vi "write16bit3DFITS.vi"(2 "u16 pixmap":u16[][][](array[numeric])=array1x300x256[76800 elements], 3 "Text":string, 4 "file path":path=path "D:/temp/fitstest.fits") -> (0 "error out":errorcluster)   [LabVIEW 2011]
panel:
  out "FITS":T1={"BITPIX"=16.0, "NAXIS"=3.0, "NAXIS1"=300.0, "NAXIS2"=300.0, "NAXIS3"=1.0, "BZERO"=0.0, "BSCALE"=1.0}
  # "OK geht mit u16 daten"
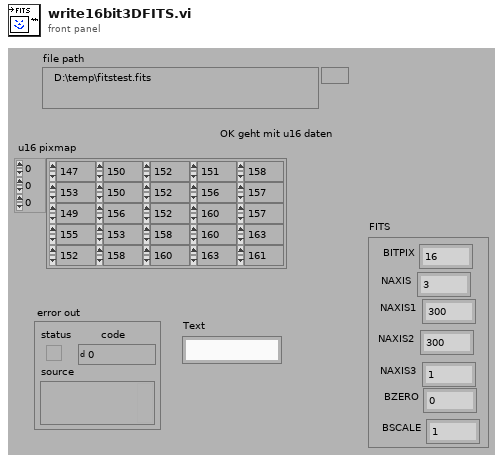
[diagram p1: front panel]
types:
  T1 = cluster{"BITPIX":sgl, "NAXIS":sgl, "NAXIS1":sgl, "NAXIS2":sgl, "NAXIS3":sgl, "BZERO":sgl, "BSCALE":sgl}
  T2 = cluster{"Tiff refnum":refnum<file>, "Byte-Reihenfolge (0:Big-Endian, 2:LSB)":enum16{"big-endian, network order", "native, host order", "little-endian"}}
  T3 = enum16{"big-endian, network order", "native, host order", "little-endian"}
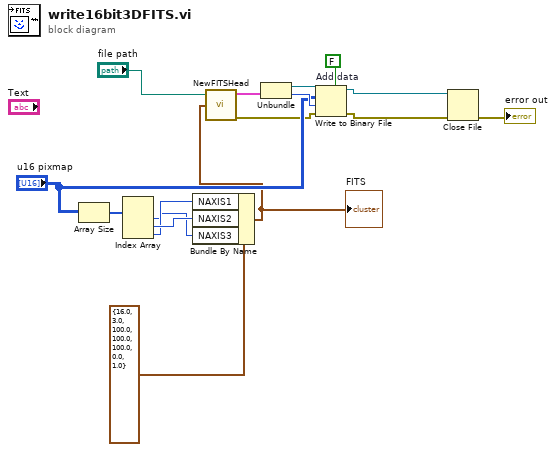
[diagram p0: block diagram]
diagram:
  n1 = Array Size(array="u16 pixmap") -> (size(s)=w14:i32[])
  n2 = Index Array(array=w14) -> (element #1=w2:i32, element #2=w12:i32, element #3=w3:i32)  [unwired: 3 in]
  n3 = Bundle By Name(cluster=T1 {"BITPIX"=16.0, "NAXIS"=3.0, "NAXIS1"=100.0, "NAXIS2"=100.0, "NAXIS3"=100.0, "BZERO"=0.0, "BSCALE"=1.0} ("FITS"), "NAXIS1"=w3, "NAXIS2"=w12, "NAXIS3"=w2) -> (w4:T1)
  "FITS" <- w4
  n4 = call "NewFITSHead.vi"("file path"="file path", "FITS"=w4) -> ("FITS file"=w11:T2, "error out"=w7:errorcluster)  [unwired: 2 in, 1 out]
  n5 = Unbundle(w11) -> ("Tiff refnum"=w10:refnum<file>, "Byte-Reihenfolge (0:Big-Endian, 2:LSB)"=w9:T3)
  n6 = Write to Binary File "Add data"(file (use dialog)=w10, data="u16 pixmap", error in=w7, 5:FALSE ("prepend array or string size? (T)"), 9:w9) -> (refnum out=w5:refnum<file>, error out=w6:errorcluster)  [unwired: 2 out]
  n7 = Close File(refnum=w5, error in=w6) -> (error out=→"error out":errorcluster)  [unwired: 1 out]
